vi "Dashboard Main.vi"() -> ()   [LabVIEW 2011]
uses:
  2012 Robot Code 2-19-12 Comp Bot/Dashboard Datatype.ctl
  <vilib>/Rock Robotics/WPI/DriverStation/WPI_DriverStationDigitalData.ctl
panel:
  in  "Harvester":bool=TRUE
  in  "Targets":bool=TRUE
  out "Lock-on":bool
  out "Manual":bool
  out "Balls in robot":dbl
  in  "Viewer":enum32{"Camera Image", "Info"}(tab)
  out "Camera Image":T1(plugin-control)
  out "Camera Image 2":T1(plugin-control)
  out "8 -- Battery":sgl(graph)
  out "Analog Input":sgl[](array[slide]) scale=0.0..5.0
  out "PWM":cluster{u8, u8}[](array[slide])=[{0, 157}, {0, 157}, {0, 157}, {0, 157}, {0, 157}, {0, 157}, {0, 157}, {0, 157}, {0, 157}, {0, 169}] scale=1.0..255.0
  out "GPIO Output Enable":bool[](array[boolean])
  out "GPIO State":bool[](array[boolean])
  out "Relay":cluster{"Forward":bool[], "Reverse":bool[]}
  out "Robot IP Address":string
  out "Shooter Speed":dbl(knob)=0.014771727831989434 scale=-1.0..1.0
  out "Left Drive":dbl(knob)=-0.010102955328711416 scale=-1.0..1.0
  out "Right Drive":dbl(knob)=-4.826648151157187e-07 scale=-1.0..1.0
  out "Distance":dbl
  out "Dashboard Datatype Warning":string="Warning: The Dashboard Datatype used by the robot project and this dashboard do not match.\nSee diagram for more details."
  out "Image Error Message":string="Timeout in Camera Communications"
  # "Analog #1"
  # "1"
  # "7"
  # "Digital #1"
  # "1"
  # "10"
  # "1"
  # "14"
  # "1"
  # "8"
  # "Communications"
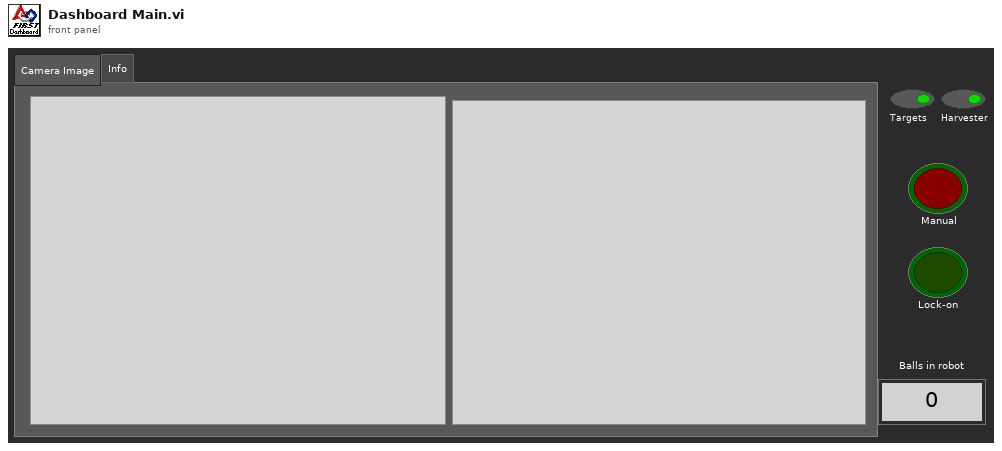
[diagram p1: front panel]
types:
  T1 = typedef "IMAQ Image.ctl" = refnum<image>
  T2 = typedef "Image Type" = u32
  T3 = typedef "Dashboard Datatype.ctl" = cluster{cluster{"AnalogModule[0]":cluster{"Channel[0]":sgl, "Channel[1]":sgl, "Channel[2]":sgl, "Channel[3]":sgl, "Channel[4]":sgl, "Channel[5]":sgl, "Channel[6]":sgl, "Channel[7]":sgl}, "AnalogModule[1]":cluster{"Channel[0]":sgl, "Channel[1]":sgl, "Channel[2]":sgl, "Channel[3]":sgl, "Channel[4]":sgl, "Channel[5]":sgl, "Channel[6]":sgl, "Channel[7]":sgl}}, cluster{"DigitalModule[0]":T4, "DigitalModule[1]":T4}, "Solenoid":u8, "Balls in robot":dbl, "Lock-on":bool, "Shooter Speed":dbl, "Right Drive":dbl, "Left Drive":dbl, "Distance":dbl, "Manual":bool}
  T4 = typedef "WPI_DriverStationDigitalData.ctl" = cluster{"Relay Fwd":u8, "Relay Rev":u8, "GPIO":u16, "GPIO_OE":u16, "PWM":cluster{"PWM[0]":u8, "PWM[1]":u8, "PWM[2]":u8, "PWM[3]":u8, "PWM[4]":u8, "PWM[5]":u8, "PWM[6]":u8, "PWM[7]":u8, "PWM[8]":u8, "PWM[9]":u8}}
  T5 = typedef "LVRectTypeDef.ctl" = cluster{"left":i16, "top":i16, "right":i16, "bottom":i16}
  T6 = cluster{"Competition mode":bool, "Robot Link":bool, "Autonomous":bool, "Enabled":bool, "E-Stop":bool}
  T7 = cluster{"AnalogModule[0]":cluster{"Channel[0]":sgl, "Channel[1]":sgl, "Channel[2]":sgl, "Channel[3]":sgl, "Channel[4]":sgl, "Channel[5]":sgl, "Channel[6]":sgl, "Channel[7]":sgl}, "AnalogModule[1]":cluster{"Channel[0]":sgl, "Channel[1]":sgl, "Channel[2]":sgl, "Channel[3]":sgl, "Channel[4]":sgl, "Channel[5]":sgl, "Channel[6]":sgl, "Channel[7]":sgl}}
  T8 = cluster{"DigitalModule[0]":T4, "DigitalModule[1]":T4}
  T9 = cluster{"Channel[0]":sgl, "Channel[1]":sgl, "Channel[2]":sgl, "Channel[3]":sgl, "Channel[4]":sgl, "Channel[5]":sgl, "Channel[6]":sgl, "Channel[7]":sgl}[]
  T10 = cluster{"Channel[0]":sgl, "Channel[1]":sgl, "Channel[2]":sgl, "Channel[3]":sgl, "Channel[4]":sgl, "Channel[5]":sgl, "Channel[6]":sgl, "Channel[7]":sgl}
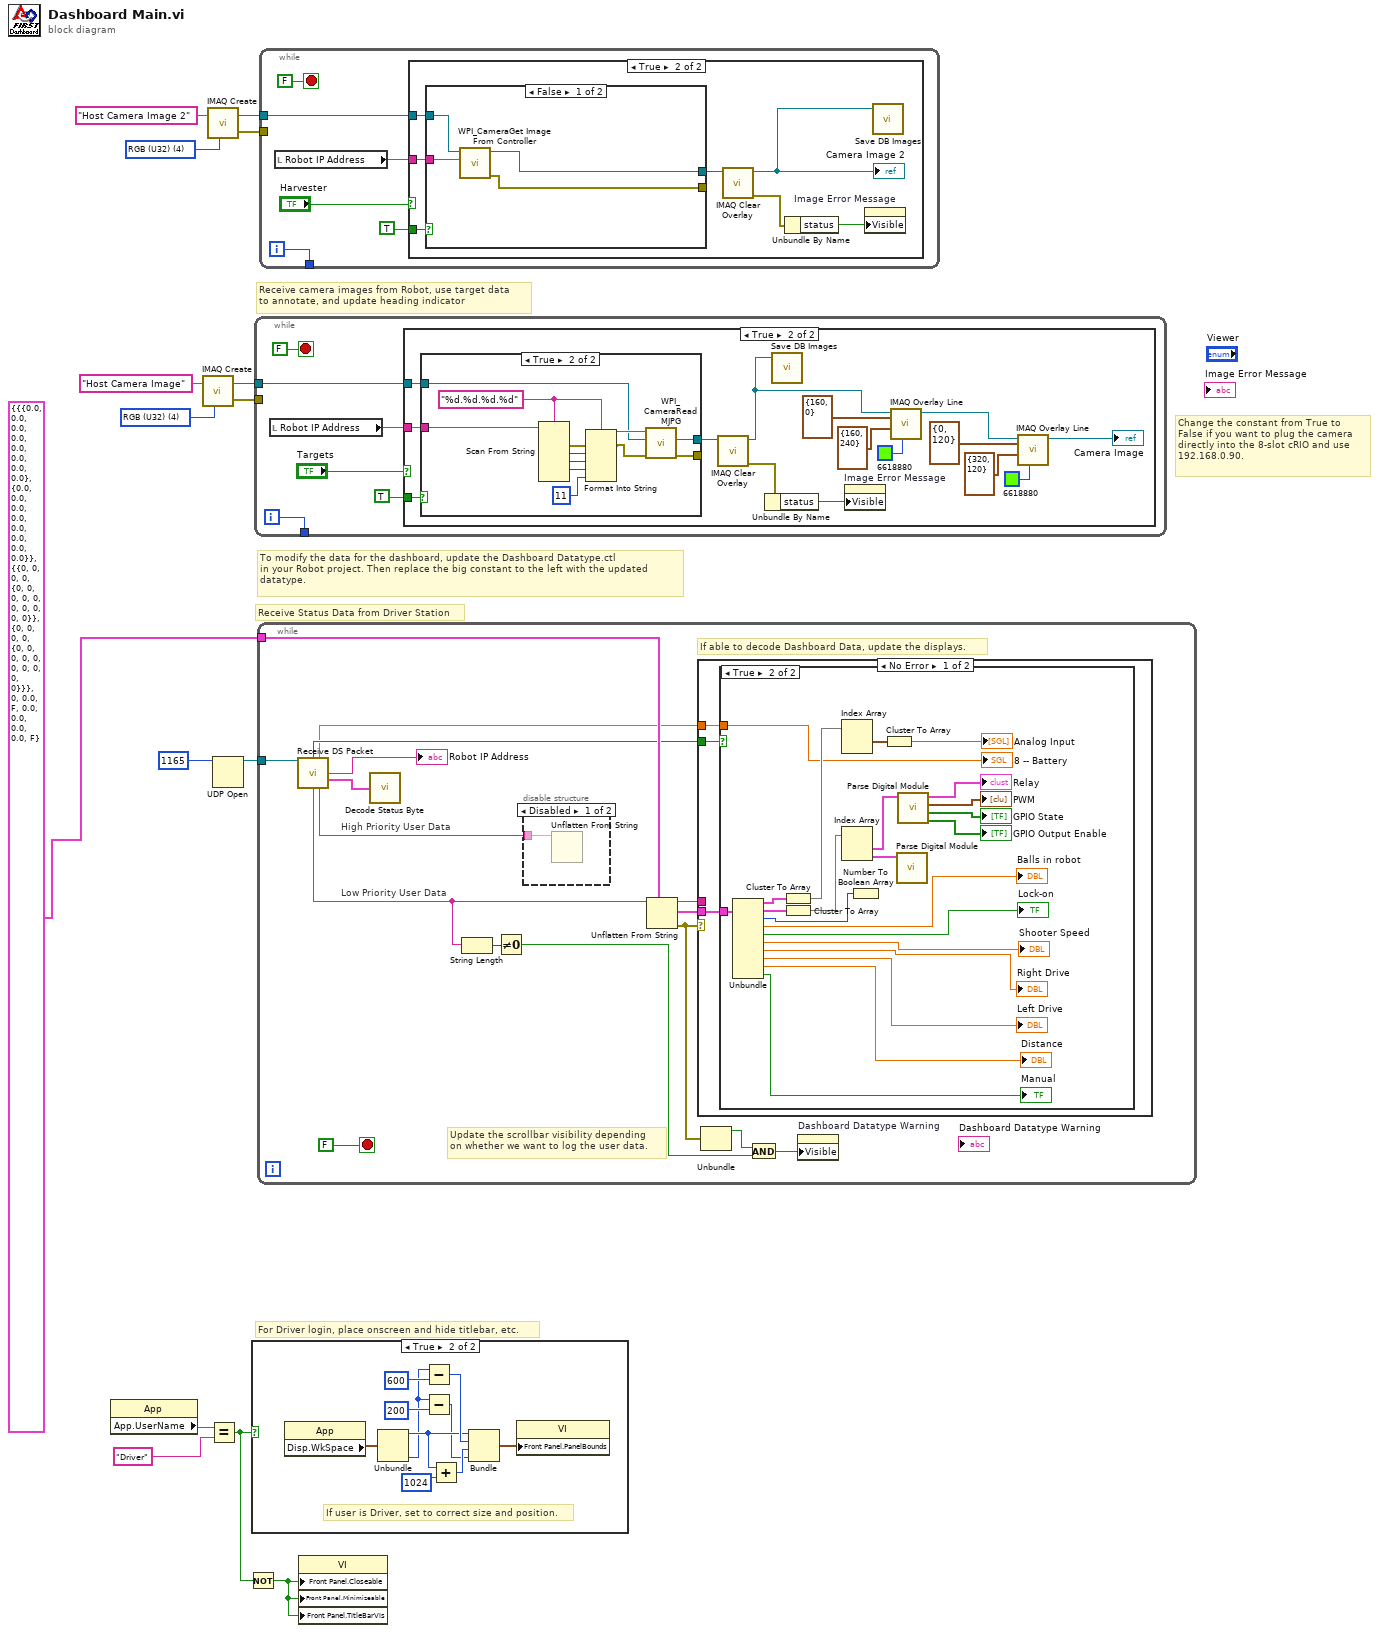
[diagram p0: block diagram]
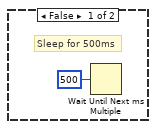
[diagram p2: hidden frame]
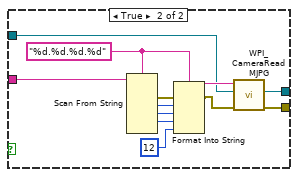
[diagram p3: hidden frame]
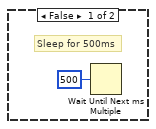
[diagram p8: hidden frame]
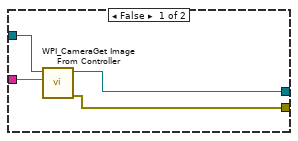
[diagram p9: hidden frame]
diagram:
  w1 = T2 4 items=["Grayscale (U8)", "Grayscale (I16)", "Grayscale (SGL)", "Complex (CSG)", "RGB (U32)", "HSL (U32)", "RGB (U64)"] ("Image Type")
  w13 = T2 4 items=["Grayscale (U8)", "Grayscale (I16)", "Grayscale (SGL)", "Complex (CSG)", "RGB (U32)", "HSL (U32)", "RGB (U64)"] ("Image Type")
  # "Change the constant from True to\nFalse if you want to plug the camera\ndirectly into the 8-slot cRIO and use\n192.168.0.90."
  # "For Driver login, place onscreen and hide titlebar, etc."
  # "To modify the data for the dashboard, update the Dashboard Datatype.ctl\nin your Robot project. Then replace the big constant to the left with the updated\ndatatype."
  # "Receive Status Data from Driver Station"
  # "Receive camera images from Robot, use target data\nto annotate, and update heading indicator"
  n1 = property class="App"() -> ("App.UserName"=w8:string)  [unwired: 2 in, 2 out]
  n2 = call "IMAQ Create"("Image Name"="Host Camera Image", "Image Type"=w13) -> ("New Image"=w11:T1, "error out"=w10:errorcluster)  [unwired: 2 in, 1 out]
  n3 = call "IMAQ Create"("Image Name"="Host Camera Image 2", "Image Type"=w1) -> ("New Image"=w3:T1, "error out"=w4:errorcluster)  [unwired: 2 in, 1 out]
  n4 = Equal?(x=w8, y="Driver") -> (x = y?=w7:bool)
  n5 = UDP Open(11:u16 1165 ("port")) -> (port=w14:refnum<k16>)  [unwired: 2 in, 4 out]
  n6 = Not(x=w7) -> (.not. x?=w6:bool)
  n7 = case shown="True" w7 {
    frame False {
    }
    frame True {
      # "If user is Driver, set to correct size and position."
      n8 = property class="App"() -> ("Disp.WkSpace"=w25:T5)  [unwired: 2 in, 2 out]
      n9 = Unbundle(w25) -> ("left"=w20:i16, "bottom"=w16:i16)  [unwired: 2 out]
      n10 = Subtract(x=w16, y=600) -> (x-y=w22:i32)
      n11 = Subtract(x=w16, y=200) -> (x-y=w17:i32)
      n12 = Add(x=w20, y=1024) -> (x+y=w21:i32)
      n13 = Bundle("left"=w20, w22, w21, w17) -> (w24:cluster{"left":i16, i32, i32, i32})  [unwired: 1 out]
      n14 = property class="VI"("Front Panel.PanelBounds"=w24) -> ()  [unwired: 2 in, 2 out]
    }
  }
  n15 = while {
    tunnel: w11 -> [w29]
    tunnel: w10 -> [_]
    tunnel: [w26] -> _
    i -> [w26]
    stop <- FALSE stop-if-true
    n16 = local read "Robot IP Address"() -> (w30:string)
    n17 = case shown="True" "Targets" {
      tunnel: w30 -> [_ w47]
      tunnel: w29 -> [_ w46]
      tunnel: TRUE -> [_ w42]
      frame False {
        # "Sleep for 500ms"
        n18 = Wait Until Next ms Multiple(millisecond multiple=u32 500) -> ()  [unwired: 1 out]
      }
      frame True {
        n19 = case shown="True" w42 {
          tunnel: w46 -> [w50 w57]
          tunnel: [w48 w55] -> _
          tunnel: [w49 w56] -> w43
          tunnel: w47 -> [w51 w60]
          frame False {
            n20 = call <vilib>:"WPI_CameraGet Image From Controller.vi"("Controller Address"=w51, "Image"=w50) -> ("error out"=w48:errorcluster, "Image Out"=w49:T1)  [unwired: 2 in, 6 out]
          }
          frame True {
            w52 = "%d.%d.%d.%d" ("format string")
            n21 = Scan From String(format string=w52, input string=w60) -> (error out=w59:errorcluster, output 1=w61:i32, output 2=w62:i32, output 3=w63:i32)  [unwired: 2 in, 7 out]
            n22 = Format Into String(format string=w52, error in=w59, w61, w62, w63, 11 ("IP Suffix:")) -> (resulting string=w58:string, error out=w54:errorcluster)  [unwired: 1 in]
            n23 = call <vilib>:"WPI_CameraRead MJPG.vi"("error in"=w54, "Image"=w57, "address"=w58) -> ("error out"=w55:errorcluster, "Image Out"=w56:T1)  [unwired: 7 in]
          }
        }
        n24 = call "IMAQ Clear Overlay"("Image"=w43) -> ("error out"=w44:errorcluster, "Image Out"=w34:T1)  [unwired: 2 in, 7 out]
        n25 = Unbundle By Name(w44) -> ("status"=w45:bool)
        n26 = call "Save DB Images.vi"("Image"=w34) -> ()  [unwired: 2 in, 1 out]
        n27 = property on="Image Error Message" class="Str"("Visible"=w45) -> ()  [unwired: 2 in, 2 out]
        n28 = call "IMAQ Overlay Line"("Color"=u32 6618880, "End Point"=cluster{"X":i32, "Y":i32} {"X"=160, "Y"=240}, "Start Point"=cluster{"X":i32, "Y":i32} {"X"=160, "Y"=0}, "Image"=w34) -> ("Image Out"=w41:T1)  [unwired: 6 in, 1 out]
        n29 = call "IMAQ Overlay Line"("Color"=u32 6618880, "End Point"=cluster{"X":i32, "Y":i32} {"X"=320, "Y"=120}, "Start Point"=cluster{"X":i32, "Y":i32} {"X"=0, "Y"=120}, "Image"=w41) -> ("Image Out"=→"Camera Image":T1)  [unwired: 6 in, 1 out]
      }
    }
  }
  n30 = while {
    tunnel: w14 -> [w77]
    tunnel: T3 {{"AnalogModule[0]"={"Channel[0]"=0.0, "Channel[1]"=0.0, "Channel[2]"=0.0, "Channel[3]"=0.0, "Channel[4]"=0.0, "Channel[5]"=0.0, "Channel[6]"=0.0, "Channel[7]"=0.0}, "AnalogModule[1]"={"Channel[0]"=0.0, "Channel[1]"=0.0, "Channel[2]"=0.0, "Channel[3]"=0.0, "Channel[4]"=0.0, "Channel[5]"=0.0, "Channel[6]"=0.0, "Channel[7]"=0.0}}, {"DigitalModule[0]"={"Relay Fwd"=0, "Relay Rev"=0, "GPIO"=0, "GPIO_OE"=0, "PWM"={"PWM[0]"=0, "PWM[1]"=0, "PWM[2]"=0, "PWM[3]"=0, "PWM[4]"=0, "PWM[5]"=0, "PWM[6]"=0, "PWM[7]"=0, "PWM[8]"=0, "PWM[9]"=0}}, "DigitalModule[1]"={"Relay Fwd"=0, "Relay Rev"=0, "GPIO"=0, "GPIO_OE"=0, "PWM"={"PWM[0]"=0, "PWM[1]"=0, "PWM[2]"=0, "PWM[3]"=0, "PWM[4]"=0, "PWM[5]"=0, "PWM[6]"=0, "PWM[7]"=0, "PWM[8]"=0, "PWM[9]"=0}}}, "Solenoid"=0, "Balls in robot"=0.0, "Lock-on"=FALSE, "Shooter Speed"=0.0, "Right Drive"=0.0, "Left Drive"=0.0, "Distance"=0.0, "Manual"=FALSE} ("Dashboard Data") -> [w76]
    stop <- FALSE stop-if-true
    # "High Priority User Data"
    # "Low Priority User Data"
    # "Update the scrollbar visibility depending\non whether we want to log the user data."
    # "If able to decode Dashboard Data, update the displays."
    n31 = call "Receive DS Packet.vi"("Recv Socket"=w77) -> ("New Dashboard Data"=w73:bool, "Battery"=w64:sgl, "Robot IP Address"=→"Robot IP Address":string, "Status"=w78:T6, "Low Priority User Data"=w66:string, "High Priority User Data"=w65:string)  [unwired: 1 in, 8 out]
    n32 = call "Decode Status Byte.vi"("Status Byte"=w78) -> ()  [unwired: 2 out]
    n33 = String Length(string=w66) -> (length=w68:i32)
    n34 = Not Equal To 0?(x=w68) -> (x != 0?=w71:bool)
    n35 = disable-structure shown="Disabled" {
      disable-tunnel: w65 -> [w80 _]
      frame Disabled {
        n36 = Unflatten From String(binary string=w80) -> ()  [unwired: 2 in, 5 out]
      }
      frame Enabled {
      }
    }
    n37 = Unflatten From String(type=w76, binary string=w66) -> (rest of the binary string=w69:string, value=w75:T3, error out=w74:errorcluster)  [unwired: 1 in, 2 out]
    n38 = case shown="No Error" w74 {
      tunnel: w75 -> [w83 _]
      tunnel: w73 -> [w82 _]
      tunnel: w69 -> [_ _]
      tunnel: w64 -> [w81 _]
      frame No Error {
        n39 = case shown="True" w82 {
          tunnel: w83 -> [_ w97]
          tunnel: w81 -> [_ w91]
          frame False {
            # "Don't update if the robot hasn't sent new data"
          }
          frame True {
            n40 = Unbundle(w97) -> (w94:T7, w95:T8, "Solenoid"=w96:u8, "Balls in robot"=→"Balls in robot":dbl, "Lock-on"=→"Lock-on":bool, "Shooter Speed"=→"Shooter Speed":dbl, "Right Drive"=→"Right Drive":dbl, "Left Drive"=→"Left Drive":dbl, "Distance"=→"Distance":dbl, "Manual"=→"Manual":bool)
            n41 = Cluster To Array(cluster=w94) -> (array=w105:T9)
            n42 = Cluster To Array(cluster=w95) -> (array=w104:T4[])
            n43 = Index Array(array=w105) -> (element #1=w92:T10)  [unwired: 2 in, 1 out]
            n44 = Index Array(array=w104) -> (element #1=w103:T4, element #2=w98:T4)  [unwired: 2 in]
            n45 = Number To Boolean Array(number=w96) -> ()  [unwired: 1 out]
            n46 = Cluster To Array(cluster=w92) -> (array=→"Analog Input":sgl[])
            n47 = call "Parse Digital Module.vi"("DigitalModule"=w98) -> ()  [unwired: 11 out]
            n48 = call "Parse Digital Module.vi"("DigitalModule"=w103) -> ("GPIO Output Enable"=→"GPIO Output Enable":bool[], "GPIO State"=→"GPIO State":bool[], "PWM"=→"PWM":cluster{u8, u8}[], "Relay"=→"Relay":cluster{"Forward":bool[], "Reverse":bool[]})  [unwired: 7 out]
            "8 -- Battery" <- w91
          }
        }
      }
      frame Error {
        # "Your datatypes don't match. The Dashboard Datatype.ctl in your Robot project\nand the big constant to the left of the loop need to match."
      }
    }
    n49 = Unbundle(w74) -> ("status"=w70:bool)  [unwired: 2 out]
    n50 = And(x=w70, y=w71) -> (x .and. y?=w72:bool)
    n51 = property on="Dashboard Datatype Warning" class="Str"("Visible"=w72) -> ()  [unwired: 2 in, 2 out]
  }
  n52 = while {
    tunnel: w3 -> [w109]
    tunnel: w4 -> [_]
    tunnel: [w107] -> _
    i -> [w107]
    stop <- FALSE stop-if-true
    n53 = local read "Robot IP Address"() -> (w110:string)
    n54 = case shown="True" "Harvester" {
      tunnel: w110 -> [_ w119]
      tunnel: w109 -> [_ w118]
      tunnel: TRUE -> [_ w113]
      frame False {
        # "Sleep for 500ms"
        n55 = Wait Until Next ms Multiple(millisecond multiple=u32 500) -> ()  [unwired: 1 out]
      }
      frame True {
        n56 = case shown="False" w113 {
          tunnel: w118 -> [w122 w129]
          tunnel: [w120 w127] -> _
          tunnel: [w121 w128] -> w115
          tunnel: w119 -> [w123 w132]
          frame False {
            n57 = call <vilib>:"WPI_CameraGet Image From Controller.vi"("Controller Address"=w123, "Image"=w122) -> ("error out"=w120:errorcluster, "Image Out"=w121:T1)  [unwired: 2 in, 6 out]
          }
          frame True {
            w124 = "%d.%d.%d.%d" ("format string")
            n58 = Scan From String(format string=w124, input string=w132) -> (error out=w131:errorcluster, output 1=w133:i32, output 2=w134:i32, output 3=w135:i32)  [unwired: 2 in, 7 out]
            n59 = Format Into String(format string=w124, error in=w131, w133, w134, w135, 12 ("IP Suffix:")) -> (resulting string=w130:string, error out=w126:errorcluster)  [unwired: 1 in]
            n60 = call <vilib>:"WPI_CameraRead MJPG.vi"("error in"=w126, "Image"=w129, "address"=w130) -> ("error out"=w127:errorcluster, "Image Out"=w128:T1)  [unwired: 7 in]
          }
        }
        n61 = call "IMAQ Clear Overlay"("Image"=w115) -> ("error out"=w116:errorcluster, "Image Out"=w114:T1)  [unwired: 2 in, 7 out]
        "Camera Image 2" <- w114
        n62 = Unbundle By Name(w116) -> ("status"=w117:bool)
        n63 = property on="Image Error Message" class="Str"("Visible"=w117) -> ()  [unwired: 2 in, 2 out]
        n64 = call "Save DB Images.vi"("Image"=w114) -> ()  [unwired: 2 in, 1 out]
      }
    }
  }
  n65 = property class="VI"("Front Panel.Closeable"=w6, "Front Panel.Minimizeable"=w6, "Front Panel.TitleBarVis"=w6) -> ()  [unwired: 2 in, 2 out]
